vi "Begin.vi"() -> (0 "error out":errorcluster)   [LabVIEW 2013]
doc: "Called before other user functions, this VI is expected to open initial I/O refnums, load in file data, and do all program initialization. Notice that the <B>error out</B> terminal is simply used for data flow. Wiring it to other structures or subVIs ensures that this VI runs first."
uses:
  <vilib>/Rock Robotics/WPI/DriverStation/WPI_DriverStationRobotMode2.ctl
  <vilib>/Rock Robotics/WPI/Joystick/WPI_JoystickDeviceEnum.ctl
  <vilib>/Rock Robotics/SystemInterfaces/DIO/FPGA_DIORelayChannel.ctl
  <vilib>/Rock Robotics/SystemInterfaces/DIO/FPGA_DIOChannel.ctl
  <vilib>/Rock Robotics/SystemInterfaces/Typedef/FPGA_TypedefDigitalModule.ctl
  <vilib>/Rock Robotics/WPI/Solenoid/WPI_SolenoidChannel.ctl
  <vilib>/Rock Robotics/SystemInterfaces/DIO/FPGA_DIOPWMChannel.ctl
  <vilib>/Rock Robotics/WPI/SafetyOutput/WPI_SafetyOutputConfigMenu.ctl
  TankDriveEnum.ctl
  PnuematicMode.ctl
  <vilib>/Rock Robotics/WPI/Camera/WPI_CameraWhite Balance Values.ctl
  <vilib>/Rock Robotics/WPI/Camera/WPI_CameraExposure Values.ctl
  <vilib>/Rock Robotics/WPI/Camera/WPI_CameraFrameRate.ctl
  <vilib>/Rock Robotics/WPI/Encoder/WPI_EncoderType.ctl
  Robot Global Data.vi
  <vilib>/Rock Robotics/WPI/Solenoid/WPI_SolenoidOpenSingle.vi
  <vilib>/Rock Robotics/WPI/RobotDrive/WPI_RobotDriveOpen4MotorWithTalon.vi
  <vilib>/Rock Robotics/WPI/Counter/WPI_CounterDigitalInputToDigitalSource.vi
  <vilib>/Rock Robotics/WPI/Compressor/WPI_CompressorGetSetRefNum.vi
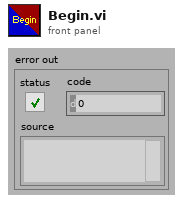
[diagram p1: front panel]
types:
  T1 = typedef "WPI_CameraFrameRate.ctl" = u32
  T2 = typedef "WPI_CameraExposure Values.ctl" = enum16{"Auto", "Flicker-free 50 Hz", "Flicker-free 60 Hz", "Hold current"}
  T3 = typedef "WPI_CameraWhite Balance Values.ctl" = enum16{"Auto", "Fixed indoor", "Fixed outdoor 1", "Fixed outdoor 2", "Fixed fluorescent 1", "Fixed fluorescent 2", "Hold current"}
  T4 = typedef "PnuematicMode.ctl" = enum16{"Init", "SetState", "Disable"}
  T5 = typedef "WPI_SolenoidChannel.ctl" = enum8{"Solenoid 1", "Solenoid 2", "Solenoid 3", "Solenoid 4", "Solenoid 5", "Solenoid 6", "Solenoid 7", "Solenoid 8", "Invalid"}
  T6 = typedef "FPGA_DIOPWMChannel.ctl" = enum8{"PWM 1", "PWM 2", "PWM 3", "PWM 4", "PWM 5", "PWM 6", "PWM 7", "PWM 8", "PWM 9", "PWM 10", "Invalid"}
  T7 = typedef "TankDriveEnum.ctl" = enum16{"Init", "LinearDrive", "SetValue", "Disable"}
  T8 = typedef "WPI_SafetyOutputConfigMenu.ctl" = enum16{"Enable", "Disable"}
  T9 = typedef "FPGA_TypedefDigitalModule.ctl" = enum16{"Digital Module 1", "Digital Module 2"}
  T10 = typedef "FPGA_DIOChannel.ctl" = enum8{"DIO 1", "DIO 2", "DIO 3", "DIO 4", "DIO 5", "DIO 6", "DIO 7", "DIO 8", "DIO 9", "DIO 10", "DIO 11", "DIO 12", "DIO 13", "DIO 14", "Invalid"}
  T11 = typedef "FPGA_DIORelayChannel.ctl" = enum8{"Relay 1", "Relay 2", "Relay 3", "Relay 4", "Relay 5", "Relay 6", "Relay 7", "Relay 8", "Invalid"}
  T12 = typedef "WPI_JoystickDeviceEnum.ctl" = enum16{"USB 1", "USB 2", "USB 3", "USB 4", "Kinect 1", "Kinect 2"}
  T13 = typedef "WPI_DriverStationRobotMode2.ctl" = enum16{"Autonomous Disabled", "Autonomous Enabled", "Teleop Disabled", "Teleop Enabled", "Timeout", "Finish", "Test Disabled", "Test Enabled"}
  T14 = typedef "WPI_EncoderType.ctl" = enum16{"1x", "2x", "4x"}
  T15 = typedef "WPI_DigitalInputDevRef.ctl" = cluster{"DevStatus":errorcluster, "DIO Channel":T10, "Digital Module":T9}
  T16 = typedef "FPGA_CounterEncoderSourceConvertionLVSourceType.ctl" = cluster{"DevStatus":errorcluster, "AnalogTriggerMode?":bool, "DigitalMode":cluster{"Digital Module":T9, "DIO Channel":T17}, "AnalogTriggerMode":cluster{"AnalogTriggerIndex":T18, "OutputType":T19}}
  T17 = typedef "FPGA_DIODigitalSourceChannel.ctl" = enum8{"DIO 1", "DIO 2", "DIO 3", "DIO 4", "DIO 5", "DIO 6", "DIO 7", "DIO 8", "DIO 9", "DIO 10", "DIO 11", "DIO 12", "DIO 13", "DIO 14", "Disabled"}
  T18 = typedef "FPGA_AnalogTriggerIndex.ctl" = enum8{"Trig 0", "Trig 1", "Trig 2", "Trig 3", "Trig 4", "Trig 5", "Trig 6", "Trig 7", "Invalid"}
  T19 = typedef "FPGA_AnalogTriggerOutType.ctl" = enum16{"InWindow", "TriggerState", "Rising", "Falling"}
  T20 = typedef "WPI_EncoderDevRef.ctl" = cluster{"DevStatus":errorcluster, "EncoderIndex":T21, "CounterIndex":T22, "DistancePerCount":dbl, "Decoding Type":T14}
  T21 = typedef "FPGA_EncoderIdx.ctl" = enum8{"Enc 0", "Enc 1", "Enc 2", "Enc 3", "Invalid"}
  T22 = typedef "FPGA_CounterCtrSystemIndex.ctl" = enum8{"Ctr 0", "Ctr 1", "Ctr 2", "Ctr 3", "Ctr 4", "Ctr 5", "Ctr 6", "Ctr 7", "Invalid"}
  T23 = typedef "WPI_SolenoidDevRef.ctl" = cluster{"DevStatus":errorcluster, "Solenoid Module":T24, "Forward Solenoid Channel":T5, "Reverse Solenoid Channel":T5}
  T24 = typedef "FPGA_TypedefSolenoidModule.ctl" = enum16{"Solenoid Module 1", "Solenoid Module 2"}
  T25 = typedef "WPI_CameraImageSize.ctl" = enum16{"640x480", "320x240", "160x120"}
  T26 = typedef "WPI_CameraDevRef.ctl" = cluster{"Camera Address":string, "CameraStatus":errorcluster, "Acquire Image Notifier":refnum<notifier>}
  T27 = typedef "WPI_RobotDriveDevRef.ctl" = cluster{"DevStatus":errorcluster, "Motors[]":T28[], "Square Inputs":bool, "Max Output":dbl, "Isochronous":bool}
  T28 = typedef "WPI_MotorControlDeviceRef.ctl" = cluster{"DeviceStatus":errorcluster, "Type":enum16{"PWM", "CAN"}, "PWM":cluster{"Digital Module":T9, "PWM Channel":T6, "DeadBand":T29}, "CAN":cluster{"Device Number":u8, "Control Mode":T30, "Semaphore":T31, "Max Vout":dbl}, "Invert":bool, "TransformRef":T32, "InvTransformRef":T32}
  T29 = typedef "WPI_PWMDeadband.ctl" = cluster{"Name":string, "maxPositivePwm":i32, "minPositivePwm":i32, "centerPwm":i32, "maxNegativePwm":i32, "minNegativePwm":i32, "angularRange":u16}
  T30 = typedef "WPI_CANJaguar_ControlMode.ctl" = enum8{"Percent VBus", "Current", "Speed", "Position", "Voltage"}
  T31 = typedef "Semaphore RefNum" = refnum<k1>
  T32 = typedef "WPI_PWMTransform_ConPane.ctl" = refnum<vi>
  T33 = typedef "WPI_JoystickDevRef.ctl" = cluster{"Device":T12}
  T34 = typedef "WPI_CompressorDevRef.ctl" = cluster{"DevStatus":errorcluster, "DigitalInputDevRef":T15, "RelayDevRef":T35}
  T35 = typedef "WPI_RelayDevRef.ctl" = cluster{"DevStatus":errorcluster, "Relay Channel":T11, "Digital Module":T9, "Relay Direction":T36}
  T36 = typedef "WPI_RelayDirection.ctl" = enum16{"Both directions", "Forward only", "Reverse only"}
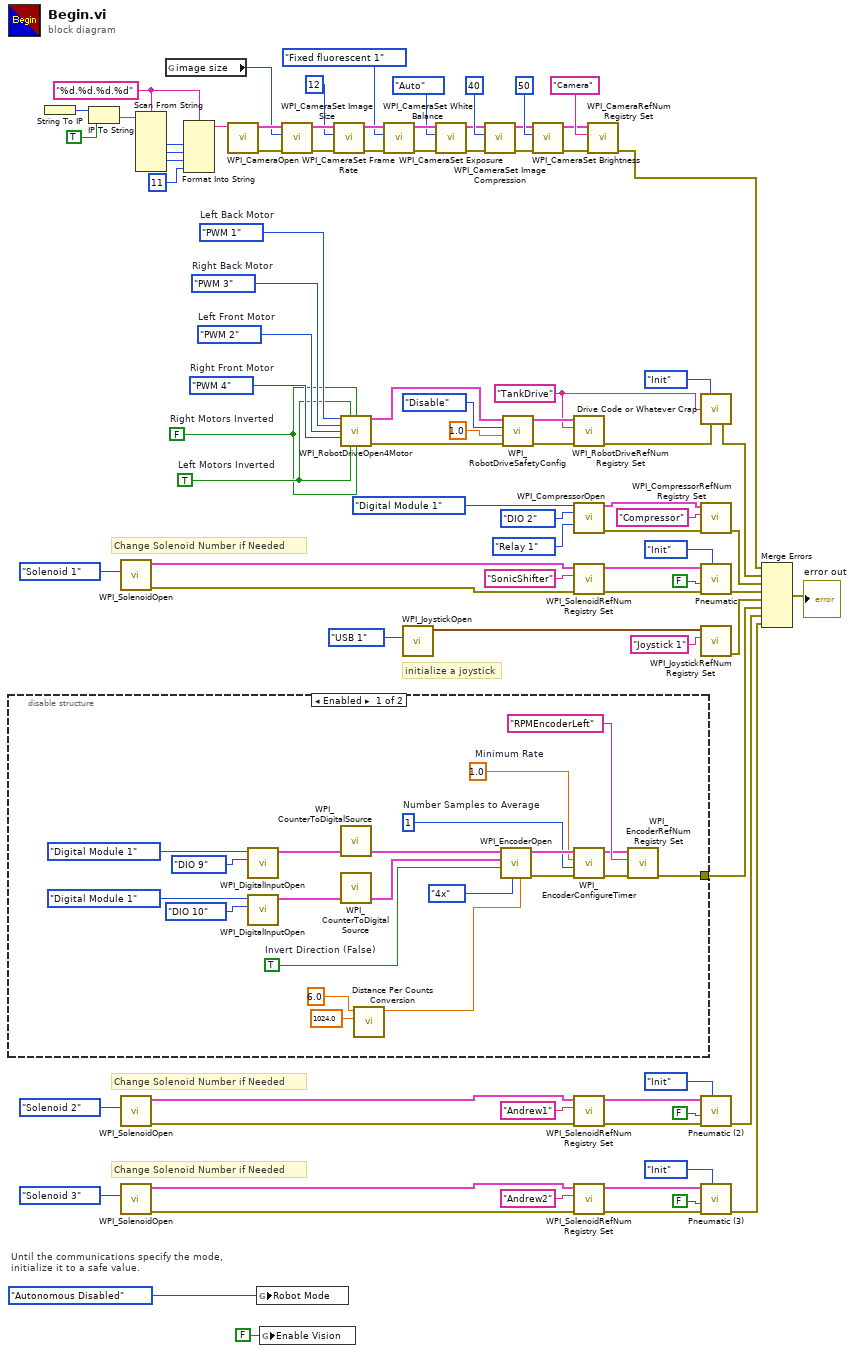
[diagram p0: block diagram]
diagram:
  w5 = "%d.%d.%d.%d" ("format string")
  w67 = FPGA_DIOPWMChannel."PWM 4"  # Right Front Motor
  w68 = FPGA_DIOPWMChannel."PWM 2"  # Left Front Motor
  w39 = "TankDrive"
  w75 = FPGA_DIOPWMChannel."PWM 3"  # Right Back Motor
  w76 = FPGA_DIOPWMChannel."PWM 1"  # Left Back Motor
  w65 = FALSE  # Right Motors Inverted
  w66 = TRUE  # Left Motors Inverted
  # "Change Solenoid Number if Needed"
  # "Change Solenoid Number if Needed"
  # "Change Solenoid Number if Needed"
  # "initialize a joystick"
  # "Until the communications specify the mode,\ninitialize it to a safe value."
  n1 = disable-structure shown="Enabled" {
    disable-tunnel: [w90 _] -> w60
    frame Enabled {
      w97 = TRUE  # Invert Direction (False)
      w99 = u8 1  # Number Samples to Average
      w100 = 1.0  # Minimum Rate
      n2 = call <vilib>:"WPI_DigitalInputOpen.vi"("DIO Channel"=FPGA_DIOChannel."DIO 9", "Digital Module (Module 1)"=FPGA_TypedefDigitalModule."Digital Module 1") -> ("DigitalInputDevRef"=w107:T15)  [unwired: 1 in, 8 out]
      n3 = call <vilib>:"WPI_DigitalInputOpen.vi"("DIO Channel"=FPGA_DIOChannel."DIO 10", "Digital Module (Module 1)"=FPGA_TypedefDigitalModule."Digital Module 1") -> ("DigitalInputDevRef"=w108:T15)  [unwired: 1 in, 8 out]
      n4 = call-poly <vilib>:"WPI_CounterToDigitalSource.vi"("DigitalInputDevRef"=w107) -> ("Digital Source"=w106:T16)  [unwired: 6 out]
      n5 = call-poly <vilib>:"WPI_CounterToDigitalSource.vi"("DigitalInputDevRef"=w108) -> ("Digital Source"=w109:T16)  [unwired: 6 out]
      n6 = call "Distance Per Counts Conversion.vi"("Counts Per Rev"=1024.0, "WheelDiameter"=6.0) -> ("Distance/Count"=w93:dbl)  [unwired: 9 in]
      n7 = call <vilib>:"WPI_EncoderOpen.vi"("DistancePerCount"=w93, "Decoding Type"=WPI_EncoderType."4x", "Invert Direction (False)"=w97, "BSource"=w109, "ASource"=w106) -> ("error out"=w95:errorcluster, "EncoderDevRef"=w103:T20)  [unwired: 3 in, 2 out]
      n8 = call <vilib>:"WPI_EncoderConfigureTimer.vi"("error in (no error)"=w95, "Number Samples to Average"=w99, "Minimum Rate"=w100, "EncoderDevRef"=w103) -> ("error out"=w94:errorcluster, "EncoderDevRef"=w96:T20)  [unwired: 6 out]
      n9 = call <vilib>:"WPI_EncoderRefNum Registry Set.vi"("error in (no error)"=w94, "refnum name"="RPMEncoderLeft", "EncoderDevRef"=w96) -> ("error out"=w90:errorcluster)  [unwired: 7 in, 1 out]
    }
    frame Disabled {
    }
  }
  n10 = String To IP() -> (0:w12:u32)  [unwired: 1 in]
  n11 = IP To String(1:TRUE ("dot notation? (F)"), 2:w12) -> (0:w10:string)
  n12 = call-poly <vilib>:"WPI_SolenoidOpen.vi"("Solenoid Channel"=WPI_SolenoidChannel."Solenoid 1") -> ("error out"=w77:errorcluster, "SolenoidDevRef"=w79:T23)  [unwired: 9 in]
  n13 = call-poly <vilib>:"WPI_SolenoidOpen.vi"("Solenoid Channel"=WPI_SolenoidChannel."Solenoid 2") -> ("error out"=w56:errorcluster, "SolenoidDevRef"=w58:T23)  [unwired: 9 in]
  n14 = call-poly <vilib>:"WPI_SolenoidOpen.vi"("Solenoid Channel"=WPI_SolenoidChannel."Solenoid 3") -> ("error out"=w53:errorcluster, "SolenoidDevRef"=w54:T23)  [unwired: 9 in]
  n15 = Scan From String(format string=w5, input string=w10) -> (output 1=w9:i32, output 2=w8:i32, output 3=w7:i32)  [unwired: 7 in, 3 out]
  n16 = global read "Robot Global Data.vi" "image size"() -> (w3:T25)
  n17 = Format Into String(format string=w5, w9, w8, w7, 11 ("Compression")) -> (resulting string=w4:string)  [unwired: 2 in, 1 out]
  n18 = call <vilib>:"WPI_CameraOpen.vi"("Camera Address"=w4) -> ("error out"=w23:errorcluster, "CameraDevRef"=w24:T26)  [unwired: 1 in, 8 out]
  n19 = global write "Robot Global Data.vi" "Robot Mode"(WPI_DriverStationRobotMode2."Autonomous Disabled" ("Robot Mode")) -> ()
  n20 = global write "Robot Global Data.vi" "Enable Vision"(FALSE ("Enable Vision")) -> ()
  n21 = call <vilib>:"WPI_CameraSet Image Size.vi"("error in (no error)"=w23, "Image Size"=w3, "CameraDevRef"=w24) -> ("error out"=w22:errorcluster, "CameraDevRef Out"=w25:T26)  [unwired: 7 out]
  n22 = call <vilib>:"WPI_CameraSet Frame Rate.vi"("error in (no error)"=w22, "Frame Rate (fps)"=T1 12, "CameraDevRef"=w25) -> ("error out"=w21:errorcluster, "CameraDevRef Out"=w27:T26)  [unwired: 7 out]
  n23 = call-poly <vilib>:"WPI_RobotDriveOpen4Motor.vi"("Rear Left Motor"=w76, "Rear Left Motor Inverted"=w66, "Rear Right Motor Inverted"=w65, "Rear Right Motor"=w75, "Front Left Motor"=w68, "Front Right Motor"=w67, "Front Left Motor Inverted"=w66, "Front Right Motor Inverted"=w65) -> ("RobotDriveDevRef"=w74:T27, "error out"=w71:errorcluster)  [unwired: 6 in]
  n24 = call <vilib>:"WPI_CameraSet White Balance.vi"("error in (no error)"=w21, "White Balance"=WPI_CameraWhite_Balance_Values."Fixed fluorescent 1", "CameraDevRef"=w27) -> ("error out"=w20:errorcluster, "CameraDevRef Out"=w26:T26)  [unwired: 7 out]
  n25 = call <vilib>:"WPI_JoystickOpen.vi"("JoystickDevice"=WPI_JoystickDeviceEnum."USB 1") -> ("JoystickDevRef"=w87:T33)  [unwired: 10 in]
  n26 = call <vilib>:"WPI_CameraSet Exposure.vi"("error in (no error)"=w20, "Exposure"=WPI_CameraExposure_Values."Auto", "CameraDevRef"=w26) -> ("error out"=w19:errorcluster, "CameraDevRef Out"=w29:T26)  [unwired: 7 out]
  n27 = call <vilib>:"WPI_CameraSet Image Compression.vi"("error in (no error)"=w19, "Compression"=40, "CameraDevRef"=w29) -> ("error out"=w18:errorcluster, "CameraDevRef Out"=w28:T26)  [unwired: 7 out]
  n28 = call <vilib>:"WPI_RobotDriveSafetyConfig.vi"("error in (no error)"=w71, "timeout (s)"=1.0, "mode"=WPI_SafetyOutputConfigMenu."Disable", "RobotDriveDevRef"=w74) -> ("error out"=w72:errorcluster, "RobotDriveDevRef"=w73:T27)  [unwired: 6 in]
  n29 = call <vilib>:"WPI_CameraSet Brightness.vi"("error in (no error)"=w18, "Brightness"=50, "CameraDevRef"=w28) -> ("error out"=w16:errorcluster, "CameraDevRef Out"=w17:T26)  [unwired: 7 out]
  n30 = call <vilib>:"WPI_RobotDriveRefNum Registry Set.vi"("error in (no error)"=w72, "refnum name"=w39, "RobotDriveDevRef"=w73) -> ("error out"=w37:errorcluster)  [unwired: 7 in, 1 out]
  n31 = call <vilib>:"WPI_CompressorOpen.vi"("Pressure Switch Digital Module (Module 1)"=FPGA_TypedefDigitalModule."Digital Module 1" ("Pressure Switch\nand Relay Module"), "Pressure Switch DIO Channel"=FPGA_DIOChannel."DIO 2" ("Pressure Switch Channel"), "Relay Channel"=FPGA_DIORelayChannel."Relay 1") -> ("CompressorDevRef"=w82:T34, "error out"=w64:errorcluster)  [unwired: 2 in, 9 out]
  n32 = call <vilib>:"WPI_SolenoidRefNum Registry Set.vi"("error in (no error)"=w77, "refnum name"="SonicShifter", "SolenoidDevRef"=w79) -> ("error out"=w51:errorcluster, "SolenoidDevRef"=w52:T23)  [unwired: 7 in]
  n33 = call <vilib>:"WPI_SolenoidRefNum Registry Set.vi"("error in (no error)"=w56, "refnum name"="Andrew1", "SolenoidDevRef"=w58) -> ("error out"=w47:errorcluster, "SolenoidDevRef"=w48:T23)  [unwired: 7 in]
  n34 = call <vilib>:"WPI_SolenoidRefNum Registry Set.vi"("error in (no error)"=w53, "refnum name"="Andrew2", "SolenoidDevRef"=w54) -> ("error out"=w43:errorcluster, "SolenoidDevRef"=w41:T23)  [unwired: 7 in]
  n35 = call <vilib>:"WPI_CameraRefNum Registry Set.vi"("error in (no error)"=w16, "refnum name"="Camera", "CameraDevRef"=w17) -> ("error out"=w2:errorcluster)  [unwired: 8 out]
  n36 = call "Drive Code or Whatever Crap.vi"("TankDriveEnum"=TankDriveEnum."Init" ("Enum"), "MotorName"=w39, "error in (no error)"=w37) -> ("error out"=w36:errorcluster)  [unwired: 10 in, 2 out]
  n37 = call <vilib>:"WPI_CompressorRefNum Registry Set.vi"("error in (no error)"=w64, "refnum name"="Compressor", "CompressorDevRef"=w82) -> ("error out"=w62:errorcluster)  [unwired: 7 in, 1 out]
  n38 = call "Pneumatic.vi"("Mode"=PnuematicMode."Init", "error in (no error)"=w51, "Default Position"=FALSE, "SolenoidDevRef"=w52) -> ("error out"=w50:errorcluster)  [unwired: 7 in]
  n39 = call <vilib>:"WPI_JoystickRefNum Registry Set.vi"("refnum name"="Joystick 1", "JoystickDevRef"=w87) -> ("error out"=w63:errorcluster)  [unwired: 8 in, 1 out]
  n40 = call "Pneumatic (2).vi"("Mode"=PnuematicMode."Init", "error in (no error)"=w47, "Default Position"=FALSE, "SolenoidDevRef"=w48) -> ("error out"=w46:errorcluster)  [unwired: 7 in]
  n41 = call "Pneumatic (3).vi"("Mode"=PnuematicMode."Init", "error in (no error)"=w43, "Default Position"=FALSE, "SolenoidDevRef"=w41) -> ("error out"=w42:errorcluster)  [unwired: 7 in]
  n42 = Merge Errors(w2, w36, w62, w50, w63, w60, w46, w42) -> (→"error out":errorcluster)
